vi "Corrections move stage + cam thesis.vi"() -> ()   [LabVIEW 2022 SP3]
uses:
  <vilib>/DAQmx/create/channels.llb/DAQmx Create Channel (CO-Pulse Generation-Time).vi
  <resource>/Zaber A Series/Zaber A Series.lvlib
  <resource>/objmgr/daqmx.rc
panel:
  in  "Number of steps":dbl
  in  "Pulse Duration":dbl=1.0 format="%.6f"
  in  "Output Terminal":tag="/Dev1/PFI12"
  in  "Counter":tag="Dev1/ctr0"
  in  "Stop":bool
  in  "Units (0: microsteps)":u16(ring) items=["microsteps", "microns", "millimeters", "inches", "degrees"]
  in  "Movement Type (0: relative)":u16(ring) items=["relative", "absolute"]
  in  "Device and Axis":string
  in  "Microstep Size (0)":dbl
  in  "Move Distance (0)":dbl format="%#_6f"
  in  "VISA resource name":refnum<visa-resource-name>
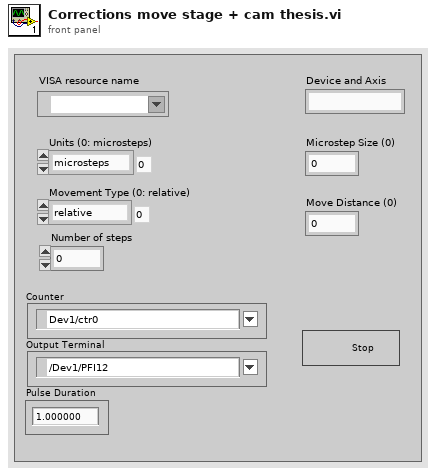
[diagram p1: front panel]
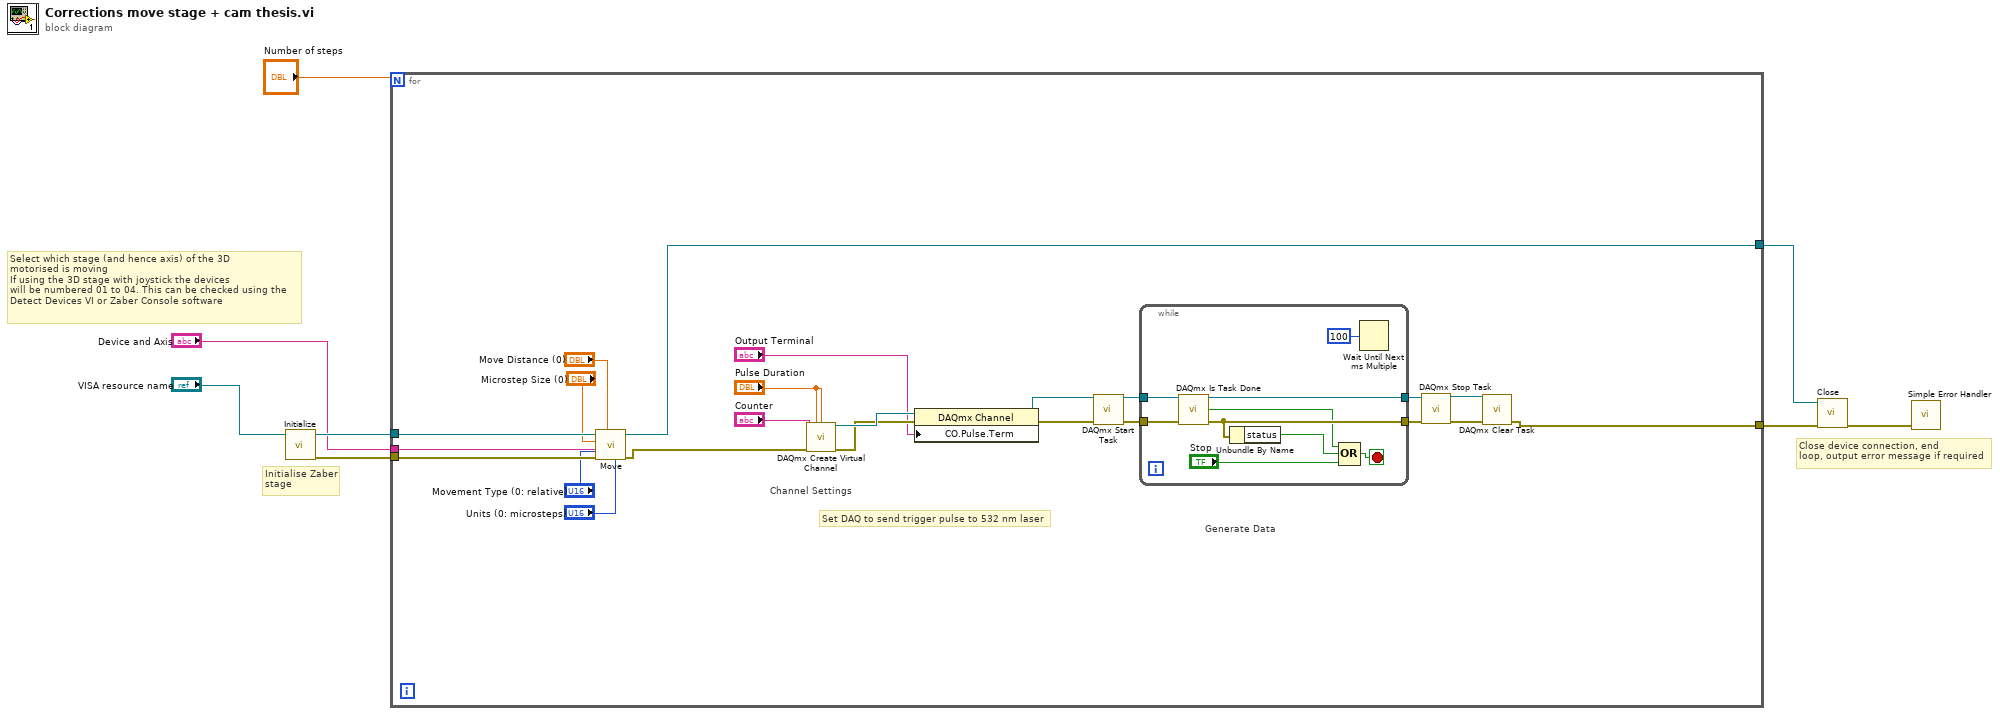
[diagram p0: block diagram]
diagram:
  # "Close device connection, end\nloop, output error message if required"
  # "Select which stage (and hence axis) of the 3D\nmotorised is moving\nIf using the 3D stage with joystick the devices\nwill be numbered 01 to 04. This can be checked using the \nDetect Devices VI or Zaber Console software"
  # "Initialise Zaber\nstage"
  n1 = call <resource>:"Initialize.vi"("VISA resource name"="VISA resource name") -> ("error out"=w6:errorcluster, "VISA resource name out"=w7:refnum<visa-resource-name>)  [unwired: 9 in]
  n2 = for {
    N: "Number of steps" -> [_]
    tunnel: w7 -> [w31]
    tunnel: w6 -> [w30]
    tunnel: "Device and Axis" -> [w27]
    tunnel: [w10] -> w4
    tunnel: [w9] -> w3
    # "Set DAQ to send trigger pulse to 532 nm laser"
    # "Generate Data"
    # "Channel Settings"
    n3 = call <resource>:"Move.vi"("Units (0: microsteps)"="Units (0: microsteps)", "Movement Type (0: relative)"="Movement Type (0: relative)", "Move Distance (0)"="Move Distance (0)", "error in (no error)"=w30, "Device and Axis"=w27, "Microstep Size (0)"="Microstep Size (0)", "VISA resource name"=w31) -> ("error out"=w11:errorcluster, "VISA resource name out"=w10:refnum<visa-resource-name>)  [unwired: 3 in]
    n4 = call-poly <vilib>:"DAQmx Create Virtual Channel.vi"("high time"="Pulse Duration", "low time"="Pulse Duration", "counter"="Counter", "error in"=w11) -> ("task out"=w21:refnum<k21>, "error out"=w20:errorcluster)  [unwired: 10 in]
    n5 = property class="DAQmx Channel"(reference=w21, error in=w20, "CO.Pulse.Term"="Output Terminal") -> (reference out=w13:refnum<k21>, error out=w12:errorcluster)
    n6 = call <vilib>:"DAQmx Start Task.vi"("task/channels in"=w13, "error in"=w12) -> ("task out"=w24:refnum<k21>, "error out"=w23:errorcluster)  [unwired: 12 in]
    n7 = while {
      tunnel: w24 -> [w40]
      tunnel: w23 -> [w39]
      tunnel: [w36] -> w16
      tunnel: [w37] -> w17
      stop <- w38 stop-if-true
      n8 = call <vilib>:"DAQmx Is Task Done.vi"("task/channels in"=w40, "error in"=w39) -> ("task out"=w37:refnum<k21>, "task done?"=w32:bool, "error out"=w36:errorcluster)  [unwired: 11 in]
      n9 = Unbundle By Name(w36) -> ("status"=w35:bool)
      n10 = Compound Arithmetic op=OR(w32, w35, "Stop") -> (w38:bool)
      n11 = Wait Until Next ms Multiple(millisecond multiple=u32 100) -> ()  [unwired: 1 out]
    }
    n12 = call <vilib>:"DAQmx Stop Task.vi"("task/channels in"=w17, "error in"=w16) -> ("task out"=w15:refnum<k21>, "error out"=w14:errorcluster)  [unwired: 12 in]
    n13 = call <vilib>:"DAQmx Clear Task.vi"("task in"=w15, "error in"=w14) -> ("error out"=w9:errorcluster)  [unwired: 13 in]
  }
  n14 = call <resource>:"Close.vi"("error in (no error)"=w3, "VISA resource name"=w4) -> ("error out"=w2:errorcluster)  [unwired: 9 in]
  n15 = call <vilib>:"Simple Error Handler.vi"("error in (no error)"=w2) -> ()  [unwired: 4 in, 5 out]
